vi "SIM Fixed-Variable Solver Select.vi"(1 "continuous integrator":T1) -> (0 "Solver Type":T2(ring))   [LabVIEW 2014]
uses:
  SIM integration method.ctl
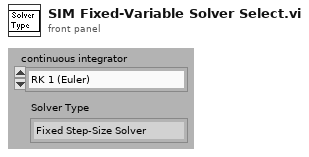
[diagram p1: front panel]
types:
  T1 = typedef "SIM integration method.ctl" = enum16{"RK 1 (Euler)", "Linearizer", "State Query", "Trim Eval", "Adams", "RK 3", "RK 4", "RK 45", "BDF", "RK 2", "RK 23", "Rosenbrock", "Discrete States Only"}
  T2 = enum16{"Fixed Step-Size Solver", "Variable Step-Size Solver"}
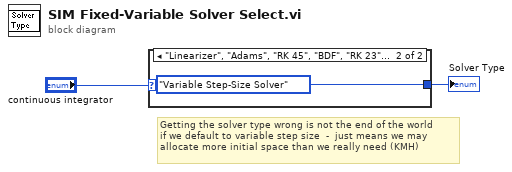
[diagram p0: block diagram]
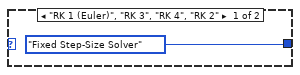
[diagram p2: hidden frame]
diagram:
  # "Getting the solver type wrong is not the end of the world\nif we default to variable step size  -  just means we may\nallocate more initial space than we really need (KMH)"
  n1 = case shown="\"Linearizer\", \"Adams\", \"RK 45\", \"BDF\", \"RK 23\", \"Rosenbrock\", Default" "continuous integrator" {
    tunnel: [T2."Fixed Step-Size Solver" ("Solver Type") T2."Variable Step-Size Solver" ("Solver Type")] -> w2
    frame "RK 1 (Euler)", "RK 3", "RK 4", "RK 2" {
    }
    frame "Linearizer", "Adams", "RK 45", "BDF", "RK 23", "Rosenbrock", Default {
    }
  }
  "Solver Type" <- w2
